vi "sample4(BasicRW All).vi"() -> ()   [LabVIEW 2011]
panel:
  out "Name/ModelNo":u16(ring) format="%04x" items=["XL320"=350, "H54-200-S500-R"=54024, "H54-100-S500-R"=53768, "H42-20-S300-R"=51200, "M54-60-S250-R"=46352, "M54-40-S250-R"=46096, "M42-10-S260-R"=43288, "L54-50-S290-R"=38176, "L54-50-S500-R"=38152, "L54-30-S400-R"=37928, "L54-30-S500-R"=37896, "L42-10-S300-R"=35072, "XM430-W350-R"=1020, "XM430-W210-R"=1030, "XH430-W350-R"=1000, "XH430-W210-R"=1010]
  in  "UPDATE":bool
  out "ACK":bool
  out "HW Error":T1
  in  "TorqueEnable":bool
  in  "OffsetTime":u32=20
  out "err":errorcluster caption="エラー出力" {"code" format="%04x"}
  in  "ID":u8=1 max=253
  in  "Baudrate":u32=57600 min=9600 max=3000000 step=100
  in  "COM":refnum<visa-resource-name> caption="COMポート"
  in  "STOP":bool
  in  "POSITION":i32(knob) min=-131594 max=131594
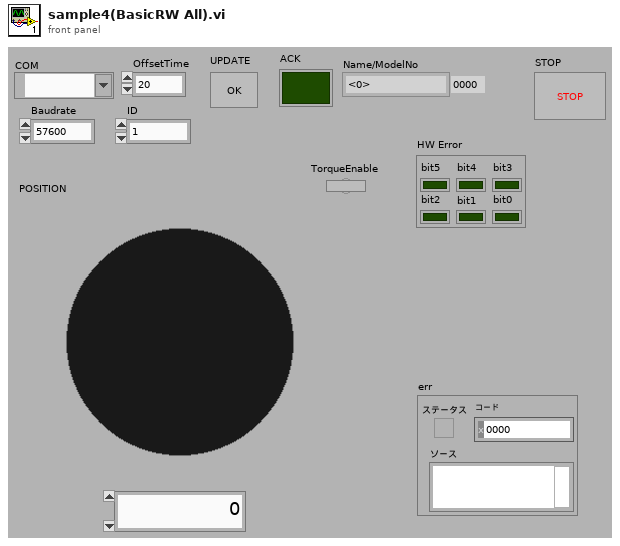
[diagram p1: front panel]
types:
  T1 = cluster{"bit0":bool, "bit1":bool, "bit2":bool, "bit3":bool, "bit4":bool, "bit5":bool}
  T2 = cluster{"Input Voltage":bool, "Motor hall sensor":bool, "Over Heating":bool, "Motor encorder":bool, "Electronical shock":bool, "Overload":bool}
  T3 = cluster{"tena":u16, "gpos":u16, "ppos":u16, "hwer":u16, "long":bool}
  T4 = cluster{"Boolean array[0]":bool, "Boolean array[1]":bool, "Boolean array[2]":bool, "Boolean array[3]":bool, "Boolean array[4]":bool, "Boolean array[5]":bool}
  T5 = cluster{"Name/ModelNo":u16, "Type":u8, "MaxPosition":i32, "MinPosition":i32, "ScaleFactor":dbl}
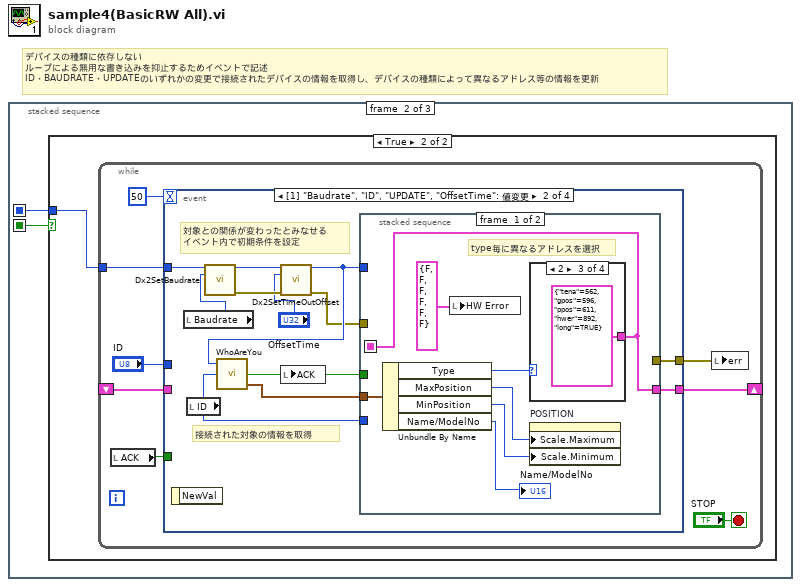
[diagram p0: block diagram]
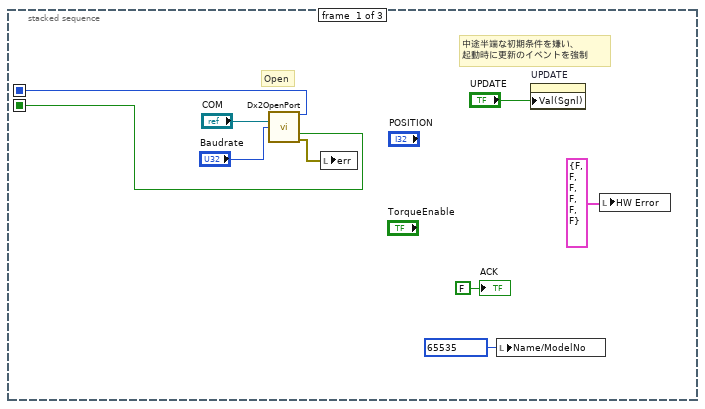
[diagram p2: hidden frame]
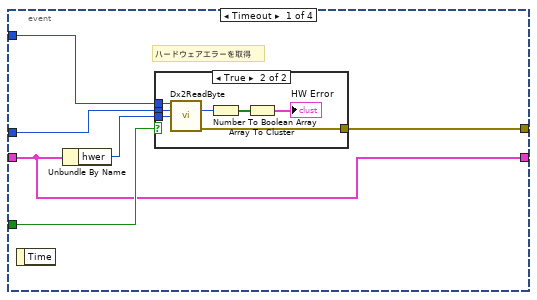
[diagram p4: hidden frame]
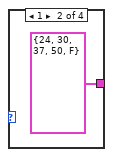
[diagram p7: hidden frame]
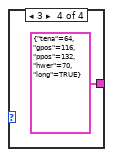
[diagram p8: hidden frame]
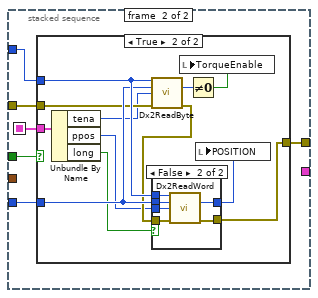
[diagram p9: hidden frame]
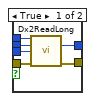
[diagram p11: hidden frame]
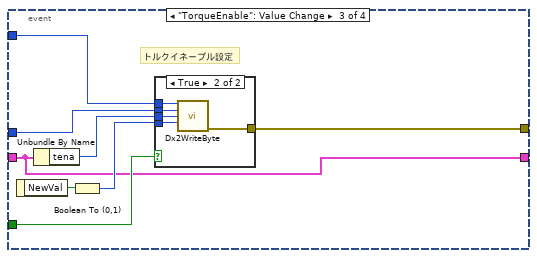
[diagram p12: hidden frame]
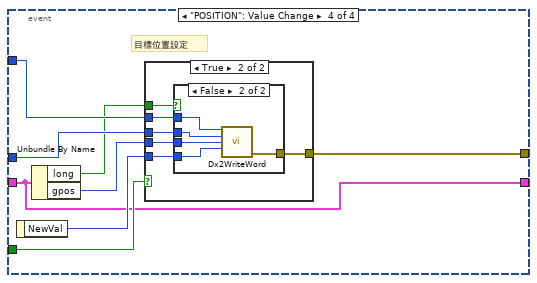
[diagram p14: hidden frame]
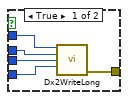
[diagram p16: hidden frame]
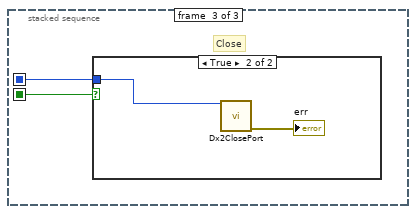
[diagram p17: hidden frame]
diagram:
  # "デバイスの種類に依存しない\nループによる無用な書き込みを抑止するためイベントで記述\nID・BAUDRATE・UPDATEのいずれかの変更で接続されたデバイスの情報を取得し、デバイスの種類によって異なるアドレス等の情報を更新"
  n1 = stacked-sequence {
    seq-local: [w7 _ _] -> [_ w11 w125]
    seq-local: [w6 _ _] -> [_ w10 w124]
    frame #0 {
      w1 = u16 65535 items=["XL320"=350, "H54-200-S500-R"=54024, "H54-100-S500-R"=53768, "H42-20-S300-R"=51200, "M54-60-S250-R"=46352, "M54-40-S250-R"=46096, "M42-10-S260-R"=43288, "L54-50-S290-R"=38176, "L54-50-S500-R"=38152, "L54-30-S400-R"=37928, "L54-30-S500-R"=37896, "L42-10-S300-R"=35072, "XM430-W350-R"=1020, "XM430-W210-R"=1030, "XH430-W350-R"=1000, "XH430-W210-R"=1010] ("Name/ModelNo")
      # "Open"
      # "中途半端な初期条件を嫌い、\n起動時に更新のイベントを強制"
      n2 = call "Dx2OpenPort.vi"("port"="COM", "baudrate"="Baudrate") -> ("dvid"=w7:u32, "成功"=w6:bool, "エラー出力"=w2:errorcluster)  [unwired: 11 in]
      n3 = local write "err"(w2) -> ()
      n4 = local write "Name/ModelNo"(w1) -> ()
      n5 = property on="UPDATE" class="Bool （指定）"("Val(Sgnl)"="UPDATE") -> ()  [unwired: 2 in, 2 out]
      n6 = local write "HW Error"(T2 {"Input Voltage"=FALSE, "Motor hall sensor"=FALSE, "Over Heating"=FALSE, "Motor encorder"=FALSE, "Electronical shock"=FALSE, "Overload"=FALSE} ("HW Error")) -> ()
      "ACK" <- FALSE ("ACK")
    }
    frame #1 {
      n7 = case shown="TRUE" w10 {
        tunnel: w11 -> [_ w12]
        frame False {
        }
        frame True {
          n8 = while {
            tunnel: w12 -> [w16]
            shift-right: [w15] -> _
            shift-left: _ -> [w14]
            stop <- "STOP" stop-if-true
            n9 = local read "ACK"() -> (w13:bool)
            n10 = event shown="[1] \"Baudrate\", \"ID\", \"UPDATE\", \"OffsetTime\": 値変更" {
              selector: _ -> [_ _ _ _]
              dyn-events: _ -> [_ _ _ _]
              timeout: 50 -> [_ _ _ _]
              tunnel: "ID" -> [w26 _ w94 w106]
              tunnel: [w23 w41 w93 w107] -> w17
              tunnel: w16 -> [w24 w45 w90 w104]
              tunnel: [w21 w40 w87 w100] -> w15
              tunnel: w14 -> [w21 _ w87 w100]
              tunnel: w13 -> [w22 _ w88 w101]
              event Timeout {
                # "ハードウェアエラーを取得"
                n11 = event-data() -> ()  [unwired: 1 in, 1 out]
                n12 = Unbundle By Name(w21) -> ("hwer"=w25:u16)
                n13 = case shown="TRUE" w22 {
                  tunnel: w26 -> [_ w33]
                  tunnel: w25 -> [_ w29]
                  tunnel: w24 -> [_ w28]
                  tunnel: [_ w27] -> w23
                  frame False {
                  }
                  frame True {
                    n14 = call "Dx2ReadByte.vi"("dvid in"=w28, "id"=w33, "address"=w29) -> ("data out"=w31:u8, "エラー出力"=w27:errorcluster)  [unwired: 9 in, 2 out]
                    n15 = Number To Boolean Array(number=w31) -> (Boolean array=w32:bool[])
                    n16 = Array To Cluster(array=w32) -> (cluster=→"HW Error":T4)
                  }
                }
              }
              event "Baudrate", "ID", "UPDATE", "OffsetTime": Value Change {
                # "接続された対象の情報を取得"
                # "対象との関係が変わったとみなせる\nイベント内で初期条件を設定"
                n17 = event-data() -> ()  [unwired: 1 in, 1 out]
                n18 = local read "Baudrate"() -> (w44:u32)
                n19 = local read "ID"() -> (w39:u8)
                n20 = call "Dx2SetBaudrate.vi"("dvid in"=w45, "Baudrate"=w44) -> ("dvid out"=w38:u32, "エラー出力"=w36:errorcluster)  [unwired: 11 in, 1 out]
                n21 = call "Dx2SetTimeOutOffset.vi"("dvid in"=w38, "OffsetTime"="OffsetTime", "エラー入力"=w36) -> ("dvid out"=w37:u32, "エラー出力"=w35:errorcluster)  [unwired: 11 in]
                n22 = call "WhoAreYou.vi"("Target ID"=w39, "dvid in"=w37) -> ("TargetInfo"=w43:T5, "matched"=w42:bool)  [unwired: 1 in, 1 out]
                n23 = local write "ACK"(w42) -> ()
                n24 = stacked-sequence {
                  seq-local: [w48 _] -> [_ w56]
                  tunnel: w43 -> [w49 _]
                  tunnel: w42 -> [_ w61]
                  tunnel: w35 -> [_ w60]
                  tunnel: [_ w59] -> w41
                  tunnel: w37 -> [_ w58]
                  tunnel: w39 -> [_ w57]
                  tunnel: [w48 _] -> w40
                  frame #0 {
                    # "type毎に異なるアドレスを選択"
                    n25 = Unbundle By Name(w49) -> ("Type"=w50:u8, "MaxPosition"=w51:i32, "MinPosition"=w52:i32, "Name/ModelNo"=→"Name/ModelNo":u16)
                    n26 = local write "HW Error"(T2 {"Input Voltage"=FALSE, "Motor hall sensor"=FALSE, "Over Heating"=FALSE, "Motor encorder"=FALSE, "Electronical shock"=FALSE, "Overload"=FALSE} ("HW Error")) -> ()
                    n27 = case shown="2" w50 {
                      tunnel: [_ T3 {"tena"=24, "gpos"=30, "ppos"=37, "hwer"=50, "long"=FALSE} T3 {"tena"=562, "gpos"=596, "ppos"=611, "hwer"=892, "long"=TRUE} T3 {"tena"=64, "gpos"=116, "ppos"=132, "hwer"=70, "long"=TRUE}] -> w48
                      frame 0, Default {
                      }
                      frame 1 {
                      }
                      frame 2 {
                      }
                      frame 3 {
                      }
                    }
                    n28 = property on="POSITION" class="Knob （指定）"("Scale.Maximum"=w51, "Scale.Minimum"=w52) -> ()  [unwired: 2 in, 2 out]
                  }
                  frame #1 {
                    n29 = case shown="TRUE" w61 {
                      tunnel: w58 -> [_ w74]
                      tunnel: w57 -> [_ w73]
                      tunnel: w60 -> [w62 w72]
                      tunnel: [w62 w70] -> w59
                      tunnel: w56 -> [_ w63]
                      frame False {
                      }
                      frame True {
                        n30 = Unbundle By Name(w63) -> ("tena"=w64:u16, "ppos"=w65:u16, "long"=w66:bool)
                        n31 = call "Dx2ReadByte.vi"("dvid in"=w74, "id"=w73, "address"=w64, "エラー入力"=w72) -> ("data out"=w69:u8, "エラー出力"=w71:errorcluster)  [unwired: 8 in, 2 out]
                        n32 = case shown="FALSE" w66 {
                          tunnel: w74 -> [w80 w86]
                          tunnel: w73 -> [w79 w85]
                          tunnel: w65 -> [w78 w84]
                          tunnel: w71 -> [w77 w83]
                          tunnel: [w76 w82] -> w70
                          tunnel: [w75 w81] -> w67
                          frame True {
                            n33 = call "Dx2ReadLong.vi"("dvid in"=w80, "id"=w79, "address"=w78, "エラー入力"=w77) -> ("data out"=w75:u32, "エラー出力"=w76:errorcluster)  [unwired: 8 in, 2 out]
                          }
                          frame False {
                            n34 = call "Dx2ReadWord.vi"("dvid in"=w86, "id"=w85, "address"=w84, "エラー入力"=w83) -> ("data out"=w81:u16, "エラー出力"=w82:errorcluster)  [unwired: 8 in, 2 out]
                          }
                        }
                        n35 = Not Equal To 0?(x=w69) -> (x != 0?=w68:bool)
                        n36 = local write "TorqueEnable"(w68) -> ()
                        n37 = local write "POSITION"(w67) -> ()
                      }
                    }
                  }
                }
              }
              event "TorqueEnable": Value Change {
                # "トルクイネーブル設定"
                n38 = event-data() -> ("NewVal"=w92:bool)  [unwired: 1 in]
                n39 = Unbundle By Name(w87) -> ("tena"=w89:u16)
                n40 = Boolean To (0,1)(Boolean=w92) -> (0, 1=w91:i16)
                n41 = case shown="TRUE" w88 {
                  tunnel: w94 -> [_ w99]
                  tunnel: [_ w98] -> w93
                  tunnel: w91 -> [_ w97]
                  tunnel: w90 -> [_ w96]
                  tunnel: w89 -> [_ w95]
                  frame False {
                  }
                  frame True {
                    n42 = call "Dx2WriteByte.vi"("dvid in"=w96, "id"=w99, "address"=w95, "data in"=w97) -> ("エラー出力"=w98:errorcluster)  [unwired: 9 in, 2 out]
                  }
                }
              }
              event "POSITION": Value Change {
                # "目標位置設定"
                n43 = event-data() -> ("NewVal"=w105:i32)  [unwired: 1 in]
                n44 = Unbundle By Name(w100) -> ("long"=w103:bool, "gpos"=w102:u16)
                n45 = case shown="TRUE" w101 {
                  tunnel: [_ w113] -> w107
                  tunnel: w106 -> [_ w112]
                  tunnel: w105 -> [_ w111]
                  tunnel: w104 -> [_ w110]
                  tunnel: w103 -> [_ w109]
                  tunnel: w102 -> [_ w108]
                  frame False {
                  }
                  frame True {
                    n46 = case shown="FALSE" w109 {
                      tunnel: [w118 w123] -> w113
                      tunnel: w110 -> [w117 w122]
                      tunnel: w112 -> [w116 w121]
                      tunnel: w111 -> [w115 w120]
                      tunnel: w108 -> [w114 w119]
                      frame True {
                        n47 = call "Dx2WriteLong.vi"("dvid in"=w117, "id"=w116, "address"=w114, "data in"=w115) -> ("エラー出力"=w118:errorcluster)  [unwired: 9 in, 2 out]
                      }
                      frame False {
                        n48 = call "Dx2WriteWord.vi"("dvid in"=w122, "id"=w121, "address"=w119, "data in"=w120) -> ("エラー出力"=w123:errorcluster)  [unwired: 9 in, 2 out]
                      }
                    }
                  }
                }
              }
            }
            n49 = local write "err"(w17) -> ()
          }
        }
      }
    }
    frame #2 {
      # "Close"
      n50 = case shown="TRUE" w124 {
        tunnel: w125 -> [_ w127]
        frame False {
        }
        frame True {
          n51 = call "Dx2ClosePort.vi"("dvid"=w127) -> ("エラー出力"=→"err":errorcluster)  [unwired: 13 in, 1 out]
        }
      }
    }
  }
